vi "Get Calibration Settings (Array).vi"(1 "Channel Settings typedef":T2[](array[typedef])) -> (0 "Calibration Settings ducktype":T1(array[cluster]))   [LabVIEW 2021, in "Settings.lvlib"]
uses:
  Settings.lvlib
  Acquisition/Channel Settings.ctl
  Acquisition/IO Device.ctl
  Acquisition/Sensor Type.ctl
  Acquisition/Acquisition.lvlib
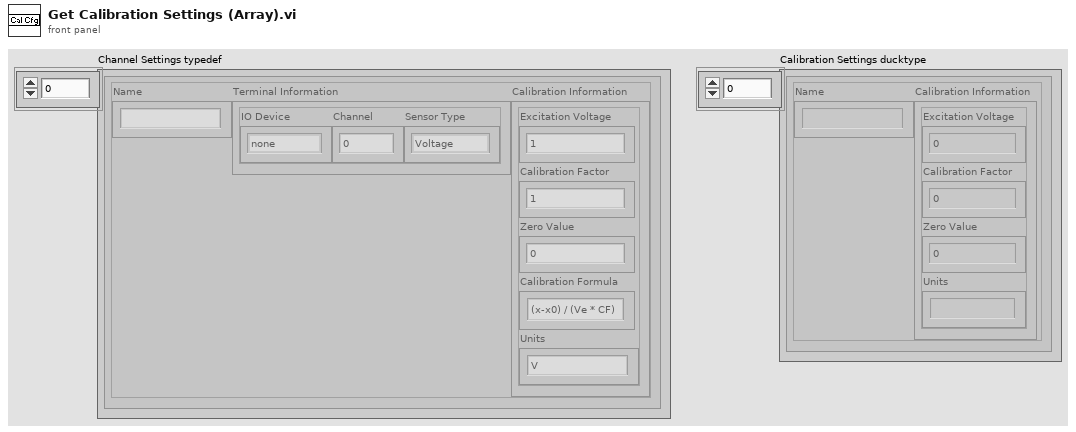
[diagram p1: front panel]
types:
  T1 = cluster{"Name":string, "Calibration Information":cluster{"Excitation Voltage":dbl, "Calibration Factor":dbl, "Zero Value":dbl, "Units":string}}[]
  T2 = typedef "Acquisition.lvlib/Channel Settings.ctl" = cluster{"Name":string, "Terminal Information":cluster{"IO Device":T3, "Channel":i32, "Sensor Type":T4}, "Calibration Information":cluster{"Excitation Voltage":dbl, "Calibration Factor":dbl, "Zero Value":dbl, "Calibration Formula":string, "Units":string}}
  T3 = typedef "Acquisition.lvlib/IO Device.ctl" = enum16{"none", "9219", "9401"}
  T4 = typedef "Acquisition.lvlib/Sensor Type.ctl" = enum16{"Voltage", "Load", "Pressure", "Encoder"}
  T5 = cluster{"Name":string, "Calibration Information":cluster{"Excitation Voltage":dbl, "Calibration Factor":dbl, "Zero Value":dbl, "Units":string}}
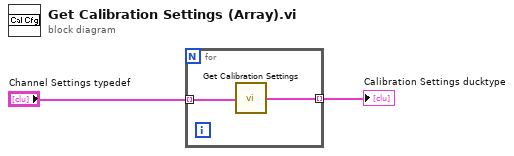
[diagram p0: block diagram]
diagram:
  n1 = for {
    tunnel: "Channel Settings typedef" -> [w4] mode=indexing
    tunnel: [w3] -> w1 mode=indexing
    n2 = call "Get Calibration Settings.vi"("Channel Settings typedef"=w4) -> ("Calibration Settings ducktype"=w3:T5)
  }
  "Calibration Settings ducktype" <- w1
